vi "variação_pressao_adq.vi"(0 "P1(mA)":dbl, 1 "P2(mA)":dbl, 2 "P3(mA)":dbl, 3 "P4(mA)":dbl, 5 "PFUNDO(mA)":dbl, 6 "JW(m/s)":dbl, 7 "JK(m/s)":dbl, 8 "Valores":T1, 9 "SIK-CV-001":bool, 11 "SIW-CV-001":bool) -> (12 "P12/L12":dbl, 13 "P34/L34":dbl, 14 "P23/L23":dbl, 15 "P2(kPa)":dbl, 16 "VALOR TEORICO":dbl, 17 "P3(kPa)":dbl, 18 "P1(kPa)":dbl, 19 "P4(kPa)":dbl, 20 "P1-P2G":bool, 21 "P2-P3R":bool, 22 "P2-P3G":bool, 23 "P1-P2R":bool, 24 "P3-P4G":bool, 25 "P3-P4R":bool, 27 "PFUNDO(kPa)":dbl)   [LabVIEW 2019]
doc: "VI destinada aos cálculos de conversão de pressões e de pressões em vazio, assim como os gradientes de pressão."
panel:
  out "Pfundo(Pa)":dbl
  out "P4(Pa)":dbl
  out "P3(Pa)":dbl
  out "P2(Pa)":dbl
  out "P1(Pa)":dbl
  # "cm/s"
  # "kPa"
  # "Pa"
  # "cm/s"
  # "kPa"
  # "Pa"
  # "kPa"
  # "Pa"
  # "kPa"
  # "Pa"
  # "kPa"
  # "Pa"
  # "MIN"
  # "MAX"
  # "P1"
  # "kPa"
  # "P2"
  # "kPa"
  # "P3"
  # "kPa"
  # "P4"
  # "kPa"
  # "Pfundo"
  # "kPa"
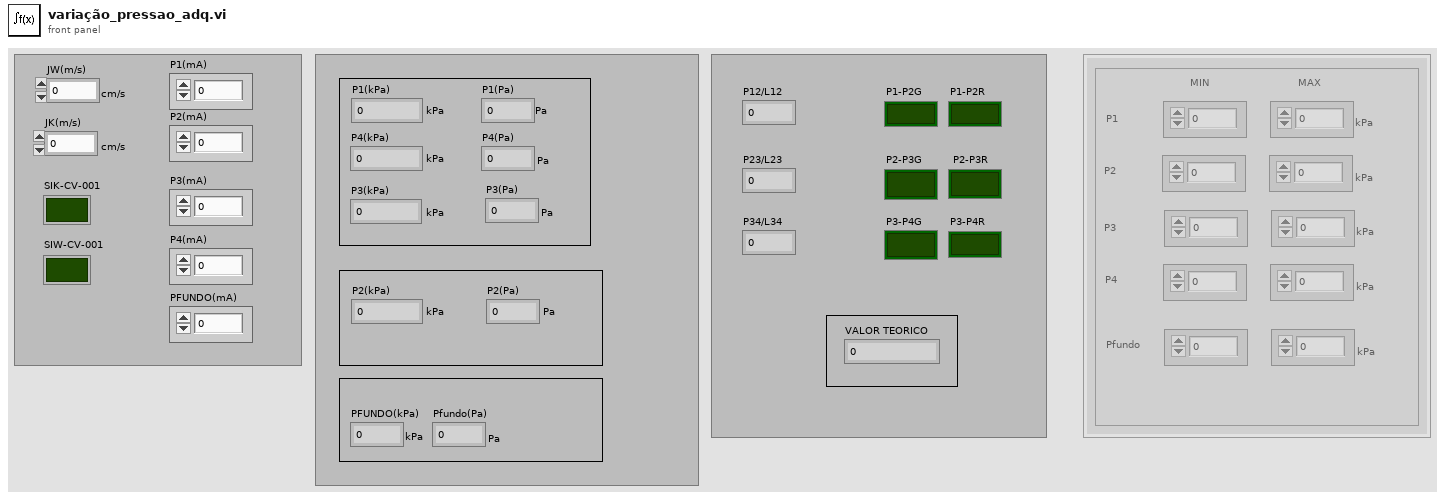
[diagram p1: front panel]
types:
  T1 = cluster{"P1 MIN":i32, "P1 MAX":i32, "P2 MIN":i32, "P2 MAX":i32, "P3 MIN":i32, "P3 MAX":i32, "P4 MIN":i32, "P4 MAX":i32, "Pfu MIN":i32, "Pfu MAX":i32}
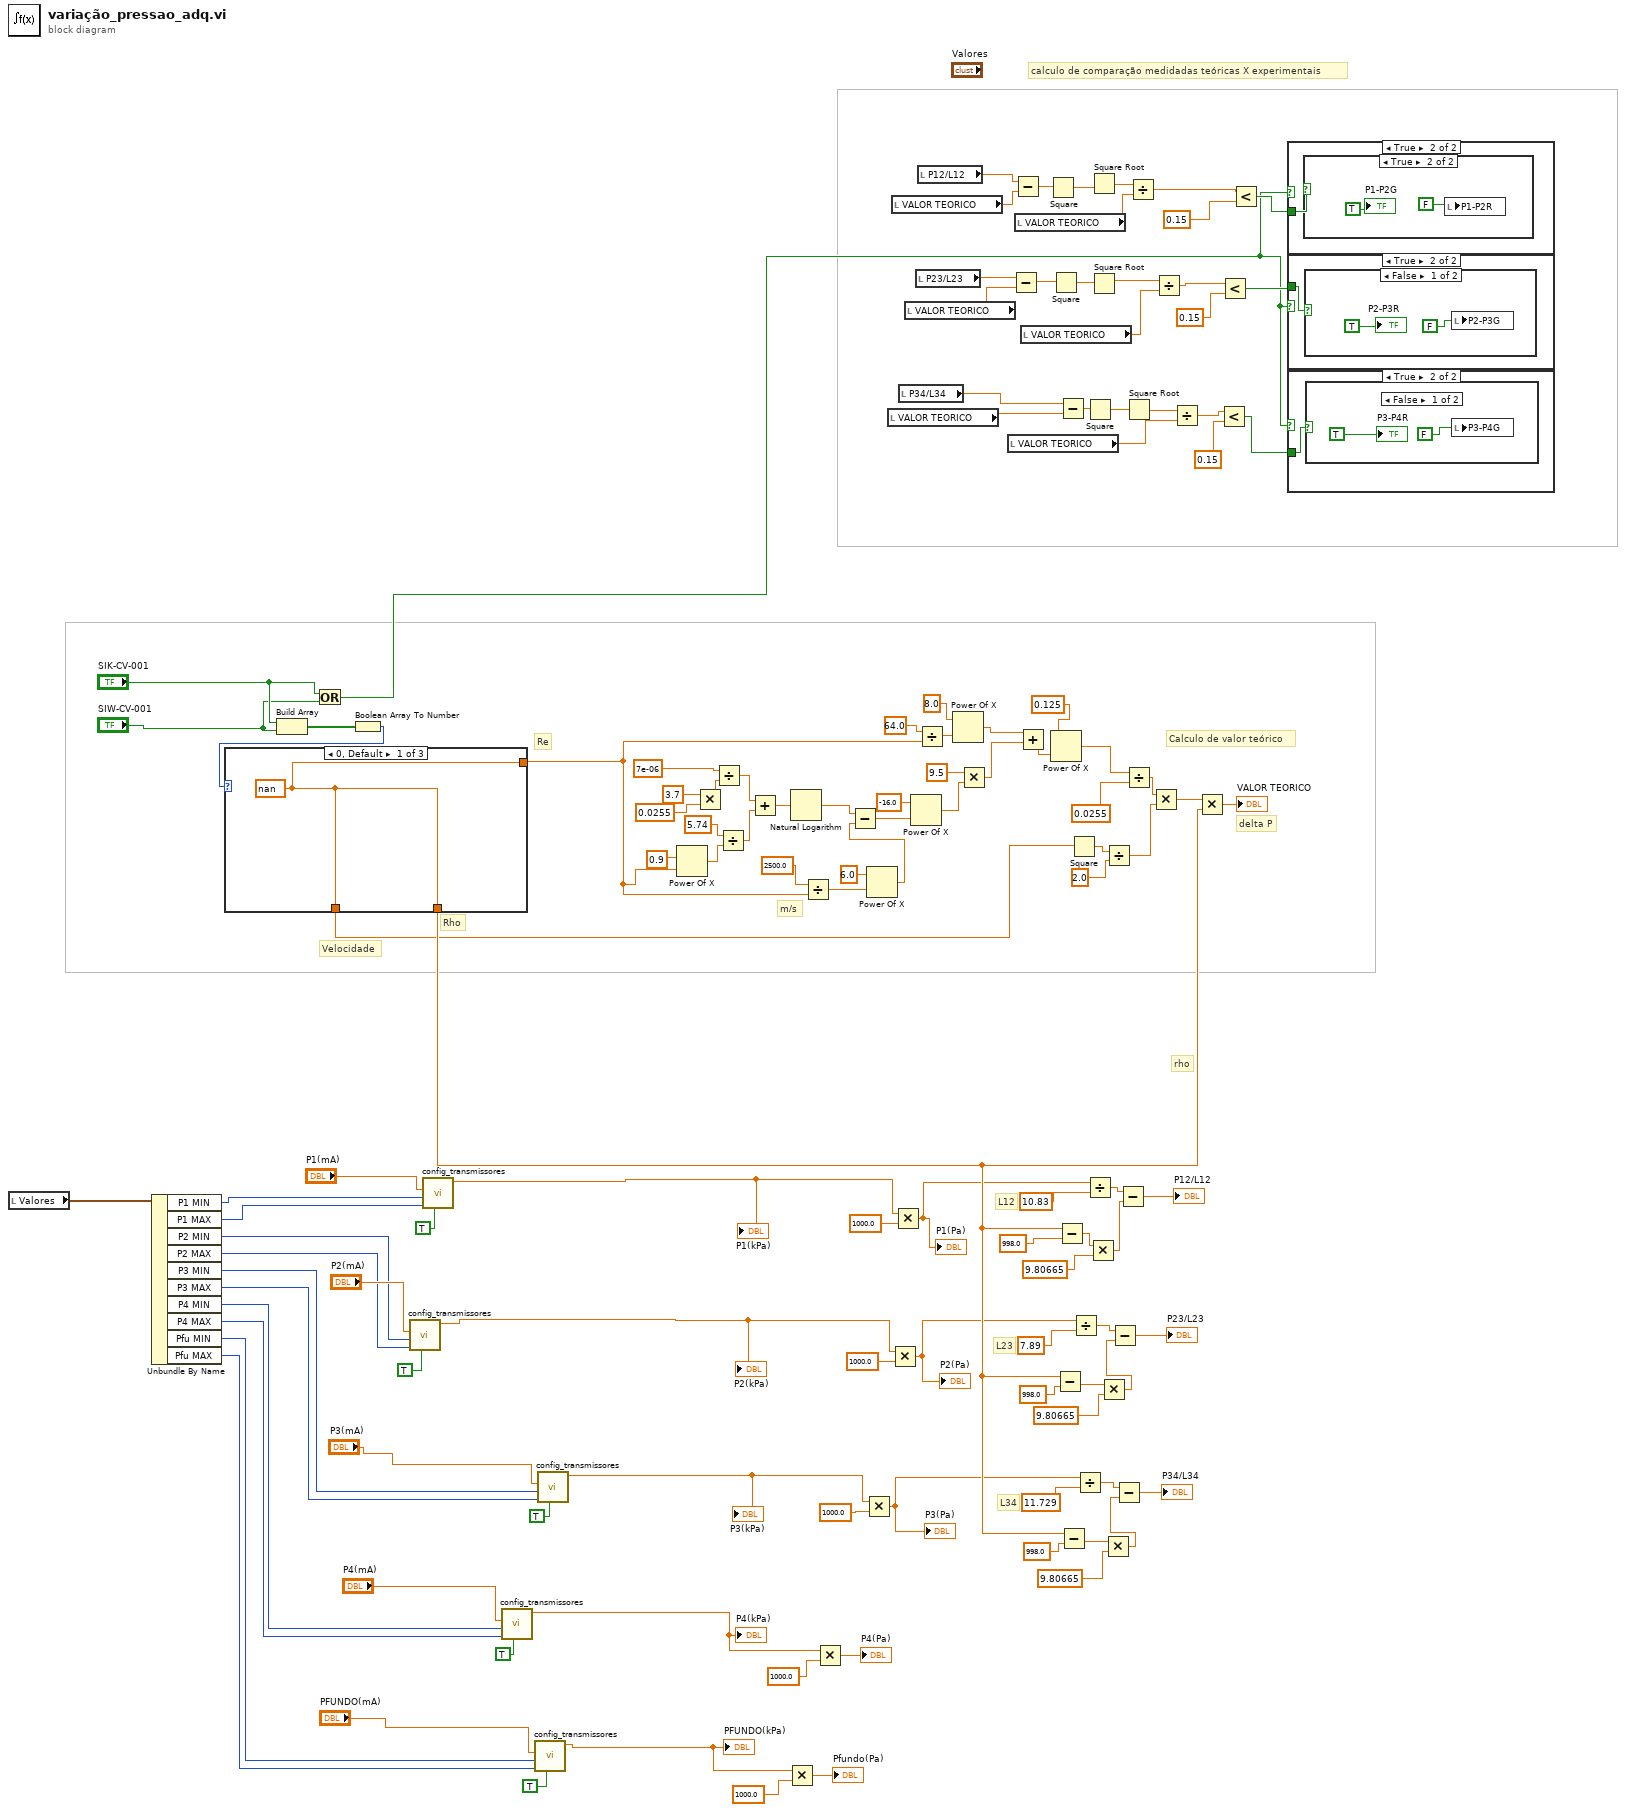
[diagram p0: block diagram]
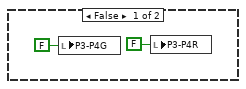
[diagram p2: hidden frame]
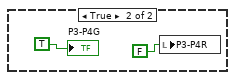
[diagram p3: hidden frame]
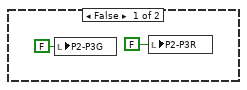
[diagram p4: hidden frame]
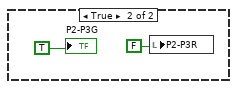
[diagram p5: hidden frame]
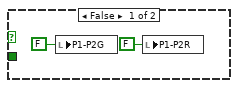
[diagram p6: hidden frame]
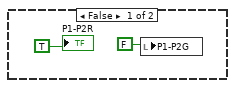
[diagram p7: hidden frame]
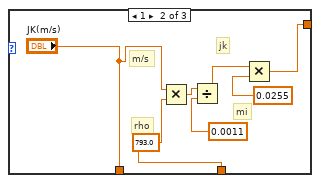
[diagram p8: hidden frame]
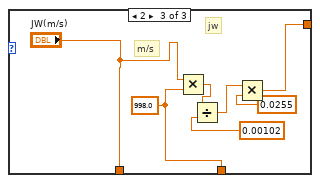
[diagram p9: hidden frame]
diagram:
  # "Calculo de valor teórico"
  # "calculo de comparação medidadas teóricas X experimentais"
  # "Velocidade"
  # "Rho"
  # "Re"
  # "m/s"
  # "delta P"
  # "L34"
  # "L23"
  # "L12"
  # "rho"
  n1 = local read "Valores"() -> (w11:T1)
  n2 = Unbundle By Name(w11) -> ("P1 MIN"=w10:i32, "P1 MAX"=w9:i32, "P2 MIN"=w8:i32, "P2 MAX"=w7:i32, "P3 MIN"=w6:i32, "P3 MAX"=w5:i32, "P4 MIN"=w4:i32, "P4 MAX"=w3:i32, "Pfu MIN"=w2:i32, "Pfu MAX"=w1:i32)
  n3 = Build Array("SIK-CV-001", "SIW-CV-001") -> (w122:bool[])
  n4 = Or(x="SIK-CV-001", y="SIW-CV-001") -> (x .or. y?=w33:bool)
  n5 = Boolean Array To Number(Boolean array=w122) -> (number=w121:u32)
  n6 = case shown="0, Default" w121 {
    tunnel: [w127 w131 w138] -> w28
    tunnel: [w127 "JK(m/s)" "JW(m/s)"] -> w30
    tunnel: [w127 w130 w137] -> w56
    frame 0, Default {
      w127 = nan
    }
    frame 1 {
      w130 = 793.0
      # "m/s"
      # "jk"
      # "rho"
      # "mi"
      n7 = Multiply(x="JK(m/s)", y=w130) -> (x*y=w134:dbl)
      n8 = Divide(x=w134, y=0.0011) -> (x/y=w132:dbl)
      n9 = Multiply(x=w132, y=0.0255) -> (x*y=w131:dbl)
    }
    frame 2 {
      w137 = 998.0
      # "m/s"
      # "jw"
      n10 = Multiply(x="JW(m/s)", y=w137) -> (x*y=w140:dbl)
      n11 = Divide(x=w140, y=0.00102) -> (x/y=w136:dbl)
      n12 = Multiply(x=w136, y=0.0255) -> (x*y=w138:dbl)
    }
  }
  n13 = call "config_transmissores.vi"("conversao corrente"=TRUE, "MAX"=w7, "MIN"=w8, "Corrente(mA)"="P2(mA)") -> ("valor"=w25:dbl)  [unwired: 7 in]
  "P2(kPa)" <- w25
  n14 = call "config_transmissores.vi"("conversao corrente"=TRUE, "MAX"=w9, "MIN"=w10, "Corrente(mA)"="P1(mA)") -> ("valor"=w26:dbl)  [unwired: 7 in]
  "P1(kPa)" <- w26
  n15 = call "config_transmissores.vi"("conversao corrente"=TRUE, "MAX"=w3, "MIN"=w4, "Corrente(mA)"="P4(mA)") -> ("valor"=w23:dbl)  [unwired: 7 in]
  "P4(kPa)" <- w23
  n16 = call "config_transmissores.vi"("conversao corrente"=TRUE, "MAX"=w1, "MIN"=w2, "Corrente(mA)"="PFUNDO(mA)") -> ("valor"=w22:dbl)  [unwired: 7 in]
  "PFUNDO(kPa)" <- w22
  n17 = call "config_transmissores.vi"("conversao corrente"=TRUE, "MAX"=w5, "MIN"=w6, "Corrente(mA)"="P3(mA)") -> ("valor"=w24:dbl)  [unwired: 7 in]
  "P3(kPa)" <- w24
  n18 = Power Of X(1:w28, 2:0.9 ("y")) -> (0:w27:dbl)
  n19 = Multiply(x=3.7, y=0.0255) -> (x*y=w114:dbl)
  n20 = Divide(x=7e-06, y=w114) -> (x/y=w112:dbl)
  n21 = Divide(x=5.74, y=w27) -> (x/y=w111:dbl)
  n22 = Add(x=w112, y=w111) -> (x+y=w110:dbl)
  n23 = Multiply(x=w22, y=1000.0) -> (x*y=→"Pfundo(Pa)":dbl)
  n24 = Natural Logarithm(1:w110) -> (0:w109:dbl)
  n25 = Divide(x=2500.0, y=w28) -> (x/y=w107:dbl)
  n26 = Multiply(x=w23, y=1000.0) -> (x*y=→"P4(Pa)":dbl)
  n27 = Multiply(x=w24, y=1000.0) -> (x*y=w49:dbl)
  "P3(Pa)" <- w49
  n28 = Power Of X(1:w107, 2:6.0 ("y")) -> (0:w105:dbl)
  n29 = Subtract(x=w109, y=w105) -> (x-y=w104:dbl)
  n30 = local read "VALOR TEORICO"() -> (w90:dbl)
  n31 = Multiply(x=w25, y=1000.0) -> (x*y=w51:dbl)
  "P2(Pa)" <- w51
  n32 = local read "VALOR TEORICO"() -> (w125:dbl)
  n33 = Multiply(x=w26, y=1000.0) -> (x*y=w38:dbl)
  "P1(Pa)" <- w38
  n34 = local read "P34/L34"() -> (w91:dbl)
  n35 = local read "VALOR TEORICO"() -> (w123:dbl)
  n36 = Power Of X(1:w104, 2:-16.0 ("y")) -> (0:w102:dbl)
  n37 = local read "P23/L23"() -> (w124:dbl)
  n38 = Divide(x=64.0, y=w28) -> (x/y=w101:dbl)
  n39 = local read "P12/L12"() -> (w126:dbl)
  n40 = Power Of X(1:w101, 2:8.0) -> (0:w99:dbl)
  n41 = Multiply(x=9.5, y=w102) -> (x*y=w119:dbl)
  n42 = local read "VALOR TEORICO"() -> (w92:dbl)
  n43 = Subtract(x=w124, y=w123) -> (x-y=w79:dbl)
  n44 = Subtract(x=w126, y=w125) -> (x-y=w81:dbl)
  n45 = local read "VALOR TEORICO"() -> (w95:dbl)
  n46 = Add(x=w99, y=w119) -> (x+y=w98:dbl)
  n47 = local read "VALOR TEORICO"() -> (w94:dbl)
  n48 = Square(x=w81) -> (x^2=w80:dbl)
  n49 = Square(x=w79) -> (x^2=w78:dbl)
  n50 = Power Of X(1:w98, 2:0.125) -> (0:w85:dbl)
  n51 = Subtract(x=w56, y=998.0) -> (x-y=w65:dbl)
  n52 = Subtract(x=w56, y=998.0) -> (x-y=w73:dbl)
  n53 = Subtract(x=w91, y=w90) -> (x-y=w77:dbl)
  n54 = Subtract(x=w56, y=998.0) -> (x-y=w60:dbl)
  n55 = Square(x=w30) -> (x^2=w88:dbl)
  n56 = Divide(x=w51, y=7.89) -> (x/y=w63:dbl)
  n57 = Divide(x=w49, y=11.729) -> (x/y=w55:dbl)
  n58 = Square(x=w77) -> (x^2=w76:dbl)
  n59 = Divide(x=w38, y=10.83) -> (x/y=w70:dbl)
  n60 = Multiply(x=w73, y=9.80665) -> (x*y=w72:dbl)
  n61 = Square Root(x=w80) -> (sqrt(x)=w96:dbl)
  n62 = Square Root(x=w78) -> (sqrt(x)=w93:dbl)
  n63 = Multiply(x=w65, y=9.80665) -> (x*y=w64:dbl)
  n64 = Multiply(x=w60, y=9.80665) -> (x*y=w61:dbl)
  n65 = Divide(x=w88, y=2.0) -> (x/y=w86:dbl)
  n66 = Subtract(x=w63, y=w64) -> (x-y=→"P23/L23":dbl)
  n67 = Subtract(x=w55, y=w61) -> (x-y=→"P34/L34":dbl)
  n68 = Subtract(x=w70, y=w72) -> (x-y=→"P12/L12":dbl)
  n69 = Square Root(x=w76) -> (sqrt(x)=w89:dbl)
  n70 = Divide(x=w85, y=0.0255) -> (x/y=w83:dbl)
  n71 = Divide(x=w96, y=w95) -> (x/y=w47:dbl)
  n72 = Multiply(x=w83, y=w86) -> (x*y=w82:dbl)
  n73 = Divide(x=w93, y=w94) -> (x/y=w44:dbl)
  n74 = Divide(x=w89, y=w92) -> (x/y=w40:dbl)
  n75 = Multiply(x=w82, y=w56) -> (x*y=→"VALOR TEORICO":dbl)
  n76 = Less?(x=w40, y=0.15) -> (x < y?=w39:bool)
  n77 = Less?(x=w44, y=0.15) -> (x < y?=w42:bool)
  n78 = Less?(x=w47, y=0.15) -> (x < y?=w45:bool)
  n79 = case shown="True" w33 {
    tunnel: w45 -> [_ w144]
    frame False {
      n80 = local write "P1-P2G"(FALSE ("P1-P2G")) -> ()
      n81 = local write "P1-P2R"(FALSE ("P1-P2R")) -> ()
    }
    frame True {
      n82 = case shown="True" w144 {
        frame False {
          n83 = local write "P1-P2G"(FALSE ("Boolean 4")) -> ()
          "P1-P2R" <- TRUE ("Boolean 4")
        }
        frame True {
          n84 = local write "P1-P2R"(FALSE ("Boolean")) -> ()
          "P1-P2G" <- TRUE ("Boolean")
        }
      }
    }
  }
  n85 = case shown="True" w33 {
    tunnel: w42 -> [_ w151]
    frame False {
      n86 = local write "P2-P3G"(FALSE ("P2-P3G")) -> ()
      n87 = local write "P2-P3R"(FALSE ("P2-P3R")) -> ()
    }
    frame True {
      n88 = case shown="False" w151 {
        frame False {
          n89 = local write "P2-P3G"(FALSE ("Boolean 5")) -> ()
          "P2-P3R" <- TRUE ("Boolean 5")
        }
        frame True {
          n90 = local write "P2-P3R"(FALSE ("Boolean 2")) -> ()
          "P2-P3G" <- TRUE ("Boolean 2")
        }
      }
    }
  }
  n91 = case shown="True" w33 {
    tunnel: w39 -> [_ w158]
    frame False {
      n92 = local write "P3-P4G"(FALSE ("P3-P4G")) -> ()
      n93 = local write "P3-P4R"(FALSE ("P3-P4R")) -> ()
    }
    frame True {
      n94 = case shown="False" w158 {
        frame False {
          n95 = local write "P3-P4G"(FALSE ("Boolean 6")) -> ()
          "P3-P4R" <- TRUE ("Boolean 6")
        }
        frame True {
          n96 = local write "P3-P4R"(FALSE ("Boolean 3")) -> ()
          "P3-P4G" <- TRUE ("Boolean 3")
        }
      }
    }
  }
